vi "TRITON_SET_CHAN_COMMAND.vi"(1 "Temperature Control Channel":i32) -> (0 "Command String":string)   [LabVIEW 2009]
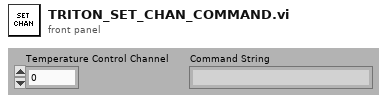
[diagram p1: front panel]
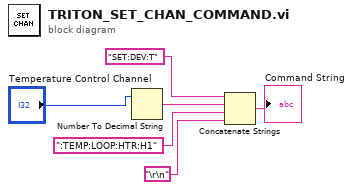
[diagram p0: block diagram]
diagram:
  n1 = Number To Decimal String(number="Temperature Control Channel") -> (decimal integer string=w4:string)  [unwired: 1 in]
  n2 = Concatenate Strings("SET:DEV:T", w4, ":TEMP:LOOP:HTR:H1", "\r\n") -> (→"Command String":string)
